vi "4~20mA 100C.vi"(1 "Numeric Indicator":dbl) -> (0 "Numeric":dbl)   [LabVIEW 2024]
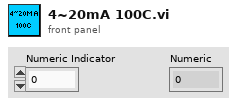
[diagram p1: front panel]
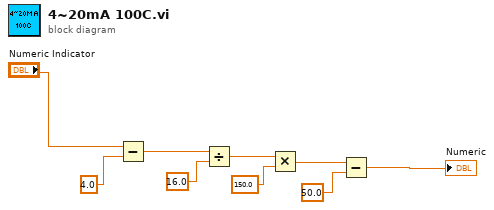
[diagram p0: block diagram]
diagram:
  n1 = Subtract(x="Numeric Indicator", y=4.0) -> (x-y=w2:dbl)
  n2 = Divide(x=w2, y=16.0) -> (x/y=w4:dbl)
  n3 = Multiply(x=w4, y=150.0) -> (x*y=w6:dbl)
  n4 = Subtract(x=w6, y=50.0) -> (x-y=→"Numeric":dbl)
